vi "SigSyn (G3)-Set Level (waveform).vi"(0 "Level":T1, 1 "Apply multiplier? (F)":bool, 2 "Name":string, 5 "Waveform in":dbl[](array[numeric]), 11 "error in (no error)":errorcluster) -> (4 "Level out":T1, 6 "Waveform out":dbl[](array[numeric]), 8 "Multiplier":dbl, 10 "Ceiling":dbl, 15 "error out":errorcluster)   [LabVIEW 2020]
uses:
  XControls/Level (G3)/Level Data.ctl
  XControls/Level (G3)/Level Units (G3).ctl
  PXI DAQ VIs/DAQ Engine VIs/PXI Globals.vi
  Utility VIs/Math VIs/dB to Linear (scalar).vi
  XControls/Level (G3)/Level (G3).xctl
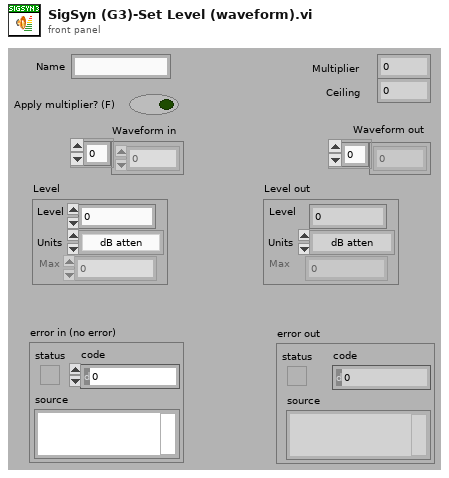
[diagram p1: front panel]
types:
  T1 = typedef "Level (G3).xctl/Level Data.ctl" = cluster{"Level":dbl, "Units":T2, "Max":dbl, "Data":cluster{"Multiplier":dbl, "Cal File":path, "Cal":cluster{"Freq (Hz)":dbl[], "Mag (dB SPL)":dbl[], "Phase (deg)":dbl[]}, "audiogram":path}}
  T2 = typedef "Level (G3).xctl/Level Units (G3).ctl" = enum16{"dB atten", "dB SPL", "dB re 1 Vrms", "dB V/Hz½", "mW", "dB HL", "Volts", "dB mW"}
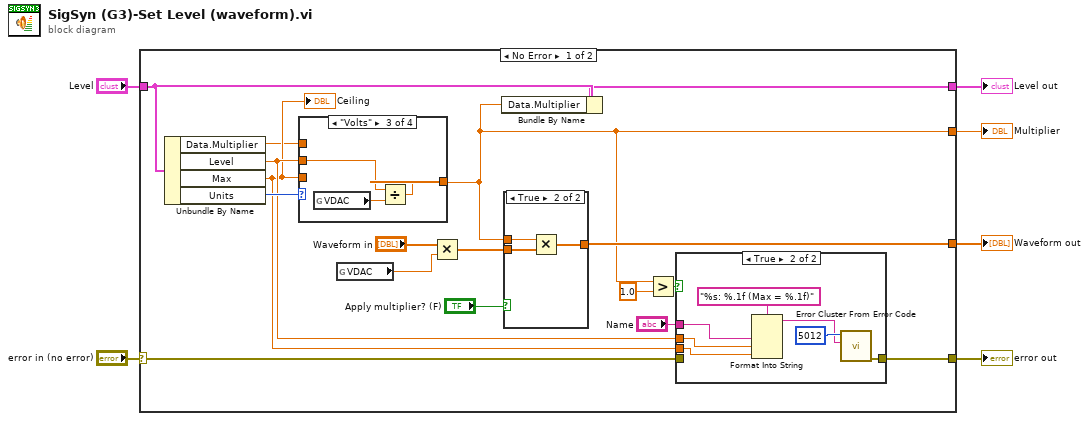
[diagram p0: block diagram]
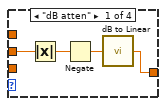
[diagram p4: hidden frame]
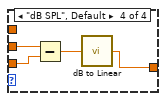
[diagram p6: hidden frame]
diagram:
  n1 = case shown="No Error" "error in (no error)" {
    selector: "error in (no error)" -> [w14 w49]
    tunnel: "Level" -> [w23 w48]
    tunnel: [w22 w48] -> w5
    tunnel: [w8 _] -> w4
    tunnel: [w21 _] -> w3
    tunnel: [w13 w49] -> w1
    frame No Error {
      n2 = Unbundle By Name(w23) -> ("Data.Multiplier"=w7:dbl, "Level"=w11:dbl, "Max"=w10:dbl, "Units"=w20:T2)
      "Ceiling" <- w10
      n3 = case shown="\"Volts\"" w20 {
        tunnel: w10 -> [_ _ _ w47]
        tunnel: w11 -> [w39 _ w42 w45]
        tunnel: [w36 w40 w41 w44] -> w8
        tunnel: w7 -> [_ w40 _ _]
        frame "dB atten" {
          n4 = Absolute Value(x=w39) -> (abs(x)=w38:dbl)
          n5 = Negate(x=w38) -> (-x=w37:dbl)
          n6 = call-poly "dB to Linear.vi"("dB"=w37) -> ("linear"=w36:dbl)
        }
        frame "mW" {
        }
        frame "Volts" {
          n7 = global read "PXI Globals.vi" "VDAC"() -> (w43:dbl)
          n8 = Divide(x=w42, y=w43) -> (x/y=w41:dbl)
        }
        frame "dB SPL", Default {
          n9 = Subtract(x=w45, y=w47) -> (x-y=w46:dbl)
          n10 = call-poly "dB to Linear.vi"("dB"=w46) -> ("linear"=w44:dbl)
        }
      }
      n11 = global read "PXI Globals.vi" "VDAC"() -> (w18:dbl)
      n12 = Multiply(x="Waveform in", y=w18) -> (x*y=w16:dbl[])
      n13 = Bundle By Name(cluster=w23, "Data.Multiplier"=w8) -> (w22:T1)
      n14 = case shown="True" "Apply multiplier? (F)" {
        tunnel: w16 -> [w32 w35]
        tunnel: w8 -> [_ w34]
        tunnel: [w32 w33] -> w21
        frame False {
        }
        frame True {
          n15 = Multiply(x=w34, y=w35) -> (x*y=w33:dbl[])
        }
      }
      n16 = Greater?(x=w8, y=1.0) -> (0:w12:bool)
      n17 = case shown="True" w12 {
        tunnel: w14 -> [w24 _]
        tunnel: [w24 w31] -> w13
        tunnel: w11 -> [_ w26]
        tunnel: w10 -> [_ w28]
        tunnel: "Name" -> [_ w25]
        frame False {
        }
        frame True {
          n18 = Format Into String(format string="%s: %.1f (Max = %.1f)", w25, w26, w28) -> (resulting string=w27:string)  [unwired: 2 in, 1 out]
          n19 = call <vilib>:"Error Cluster From Error Code.vi"("error message (\"\")"=w27, "error code (0)"=5012) -> ("error out"=w31:errorcluster)  [unwired: 7 in]
        }
      }
    }
    frame Error {
    }
  }
  "error out" <- w1
  "Waveform out" <- w3
  "Level out" <- w5
  "Multiplier" <- w4
